vi "Decay Plot.vi"() -> ()   [LabVIEW 2015]
uses:
  <vilib>/Platform/TimedLoop/XDataNode/timing_clust.ctl
  <vilib>/Platform/TimedLoop/XDataNode/nitl_modes.ctl
  <vilib>/Platform/TimedLoop/XDataNode/wakeup.ctl
  <vilib>/Utility/file.llb/Write Delimited Spreadsheet (DBL).vi
  <vilib>/platform/TimedLoop/XDataNode/XDataNode.xnode
  <vilib>/Platform/TimedLoop/XDataNode/XDNodeRunTimeDep.lvlib
panel:
  in  "Acquisition Time [s]":dbl
  in  "Period[s]":dbl
  in  "stop":bool
  out "counts per period":dbl(knob) scale=0.0..100.0
  in  "File to Save":path
  out "Waveform Graph":waveform(i32)(graph)={"t0"=timestamp(0 s since 1904-01-01), "dt"=1.0, "Y"=[0, 87, 72, 86, 74, 71, 79, 82, 78, 87, 69, 82, 59, 72, 68, 69, 61, 61, 63, 73, 74, 62, 72, 68, 70, 80, 63, 55, 66, 44, 55, 54, 64, 73, 64, 51, 68, 59, 61, 70, 55, 55, 56, 52, 69, 48, 56, 64, 49, 64, 57, 58, 40, 42, 36, 42, 56, 64, 57, 41, 60, 54, 39, 46, 41, 50, 41, 56, 33, 51, 55, 43, 49, 42, 38, 49, 48, 50, 40, 51, 40, 35, 40, 43, 35, 39, 40, 34, 35, 43, 43, 34, 39, 32, 39, 32, 30, 41, 34, 35, 40, 31, 28, 36, 39, 39, 31, 28, 32, 26, 27, 22, 28, 29, 22, 32, 31, 34, 29, 27, 31, 30, 26, 32, 23, 28, 23, 31, 32, 30, 36, 20, 16, 34, 27, 20, 24, 31, 30, 21, 30, 21, 27, 26, 24, 22, 21, 19, 24, 33, 20, 23, 24, 22, 17, 19, 27, 22, 17, 23, 19, 10, 21, 12, 17, 14, 21, 13, 26, 30, 17, 18, 22, 15, 18, 14, 13, 14, 22, 19, 15, 13, 23, 21, 19, 17, 15, 18, 12, 11, 15, 13, 17, 21, 20, 16, 18, 12, 14, 14, 16, 14, 24, 12, 14, 9, 18, 16, 11, 11, 13, 17, 11, 10, 7, 20, 14, 16, 14, 13, 12, 12, 10, 13, 17, 19, 13, 17, 15, 9, 11, 5, 14, 13, 16, 12, 11, 7, 11, 11, 9, 11, 10, 11, 11, 12, 9, 12, 9, 10, 8, 11, 12, 13, 11, 8, 11, 12, 9, 4, 12, 9, 11, 6, 10, 8, 10, 9, 13, 10, 11, 5, 14, 11, 13, 10, 5, 8, 11, 9, 6, 5, 4, 11, 6, 9, 10, 10, 11, 9, 6, 9, 7, 8, 9, 12, 11, 8, 11, 7, 12]}
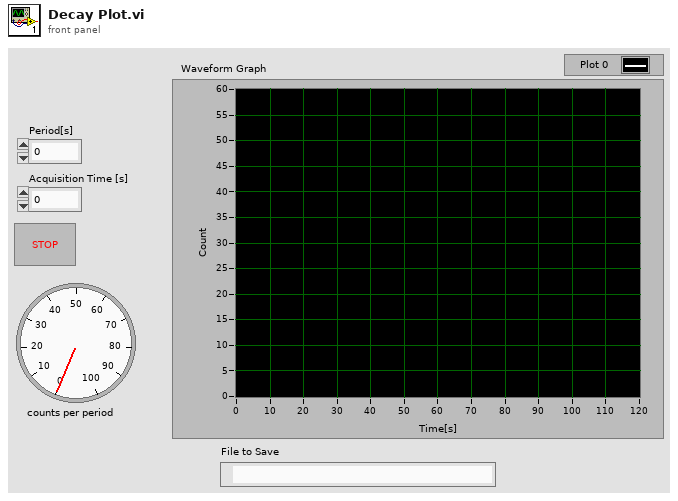
[diagram p1: front panel]
types:
  T1 = typedef "XDNodeRunTimeDep.lvlib/timing_clust.ctl" = cluster{"Expected End [f-1]":u64, "Actual End [f-1]":u64, "Finished Late? [f-1]":bool, "Expected End [i-1]":u64, "Actual End [i-1]":u64, "Finished Late? [i-1]":bool, "Expected Start [i]":u64, "Actual Start [i]":u64, "Expected Start [f]":u64, "Actual Start [f]":u64, "Source Name":string, "Structure Name":string, "Period":i64, "Deadline":i64, "Offset":i64, "Start":i64, "Priority":i32, "Timeout":i32, "Mode":T2, "Wakeup Reason":T3, "Error":errorcluster, "Source Type":string, "Secondary Source Type":string, "Global End Time":u64, "Global Start Time":u64, "Frame Duration":u64, "Iteration Duration":u64, "Assigned CPU":i32, "I/O Scan Engine Mode":u32}
  T2 = typedef "XDNodeRunTimeDep.lvlib/nitl_modes.ctl" = enum32{"No Change", "Process missed periods, maintain original phase", "Discard missed periods, maintain original phase", "Process missed periods, ignore original phase", "Discard missed periods, ignore original phase"}
  T3 = typedef "XDNodeRunTimeDep.lvlib/wakeup.ctl" = enum32{"Normal", "Aborted", "Asynchronous wakeup", "Timing source error", "Timed loop error", "Timeout"}
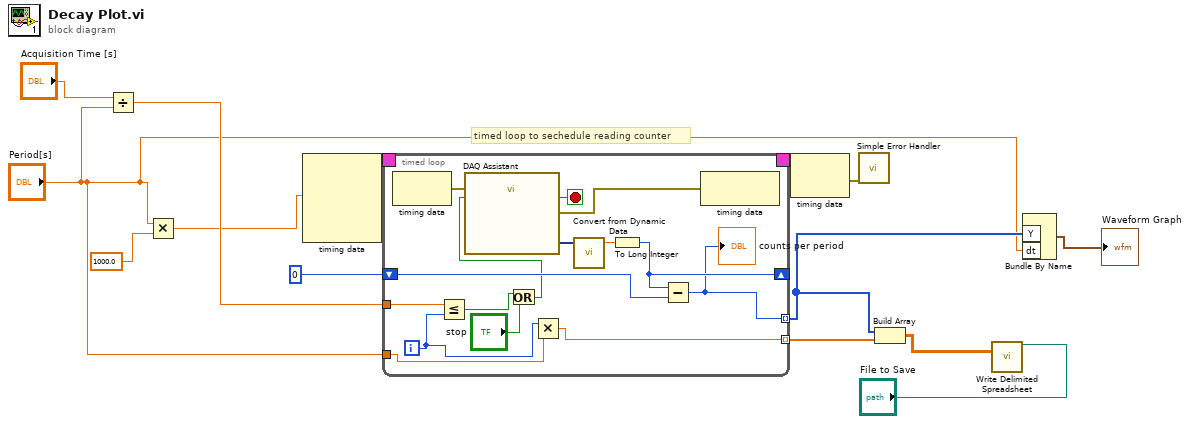
[diagram p0: block diagram]
diagram:
  # "timed loop to sechedule reading counter"
  n1 = Divide(x="Acquisition Time [s]", y="Period[s]") -> (x/y=w6:dbl)
  n2 = Multiply(x="Period[s]", y=1000.0) -> (x*y=w5:dbl)
  n3 = node-c288(w5) -> (w10:T1)  [unwired: 3 in]
  n4 = timed-loop {
    timing: w10 -> [_]
    timing-out: [_] -> w9
    shift-right: [w19] -> _
    shift-left: 0 -> [w28]
    tunnel: w6 -> [w23]
    tunnel: [w18] -> w4 mode=indexing
    tunnel: "Period[s]" -> [w16]
    tunnel: [w15] -> w2 mode=indexing
    i -> [w17]
    stop <- w27 stop-if-true
    n5 = node-c288() -> (w24:errorcluster)  [unwired: 1 in]
    n6 = Less Or Equal?(x=w23, y=w17) -> (x <= y?=w22:bool)
    n7 = Or(x=w22, y="stop") -> (x .or. y?=w20:bool)
    n8 = call "DAQ Assistant"("error in"=w24, "stop (F)"=w20) -> ("data"=w29:dynamicdata, "stopped"=w27:bool, "error out"=w25:errorcluster)  [unwired: 14 in, 1 out]
    n9 = Multiply(x=w17, y=w16) -> (x*y=w15:dbl)
    n10 = call "Convert from Dynamic Data"("Dynamic Data Type"=w29) -> ("Scalar"=w26:dbl)  [unwired: 3 in]
    n11 = To Long Integer(number=w26) -> (32bit integer=w19:i32)
    n12 = Subtract(x=w19, y=w28) -> (x-y=w18:i32)
    "counts per period" <- w18
    n13 = node-c288(w25) -> ()  [unwired: 1 out]
  }
  n14 = node-c288(w9) -> (w8:errorcluster)
  n15 = call <vilib>:"Simple Error Handler.vi"("error in (no error)"=w8) -> ()  [unwired: 4 in, 5 out]
  n16 = Build Array(w4, w2) -> (w3:dbl[][])
  n17 = call-poly <vilib>:"Write Delimited Spreadsheet.vi"("file path (dialog if empty)"="File to Save", "2D data"=w3) -> ()  [unwired: 12 in, 2 out]
  n18 = Bundle By Name("Y"=w4, "dt"="Period[s]") -> (→"Waveform Graph":waveform(i32))  [unwired: 1 in]
